vi "FFTdB&Phase_row_Ch3.vi"(8 "Freq. Step (Hz) (for Display here only)":dbl=1.0 format="%.2f", 9 "Sample Period (ms)":dbl=0.032 format="%.6f", 10 "Array Row (0base)":i16=1 min=0 max=3 step=1, 11 "Array IN":dbl[][](array[numeric]) format="%.2f") -> (0 "Phase(Radians)DataOut":dbl[](array[numeric]) format="%.2f", 1 "Magnitude( RMS dB) DataOut":dbl[](array[numeric]) format="%.2f", 2 "Magnitude (RMS dB) Plot":cluster{"Array":dbl[], "Unwrapped Phase":dbl[]}(graph), 3 "WaveformDataOut":dbl[](array[numeric]) format="%.2f", 4 "Phase (radians) Plot":cluster{"Array":dbl[], "Unwrapped Phase":dbl[]}(graph), 5 "Waveform Plot":cluster{i32, dbl, dbl[]}(graph)={0, 0.032, []})   [LabVIEW 2015]
panel:
  # "Freq. Step isn't needed if the FFT outputs are used but  the FFT-Plot outputs are not used"
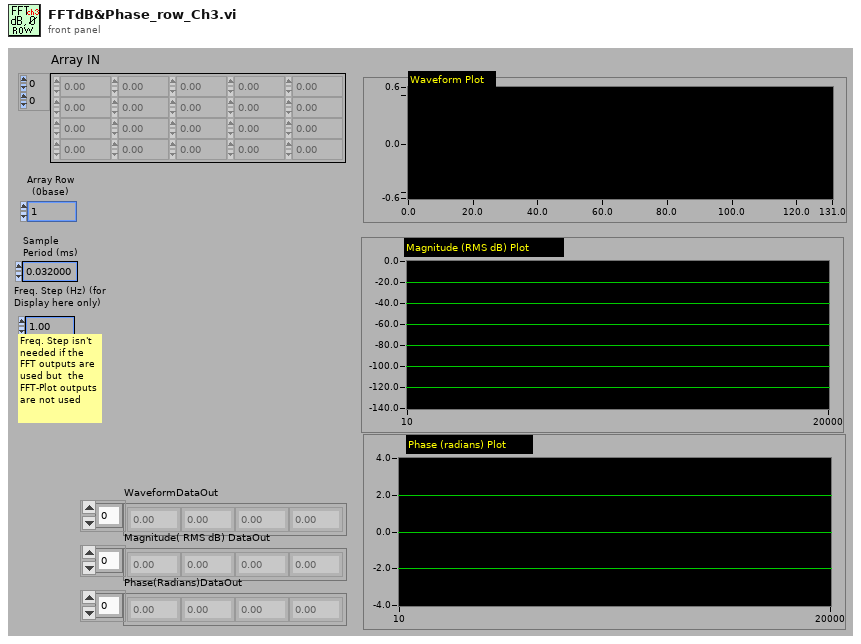
[diagram p1: front panel]
types:
  T1 = cluster{i32, "Sample Period (ms)":dbl, "Array IN":dbl[]}
  T2 = cluster{"Array":dbl[], "+Freq. Mag of FFT (dB rms)":dbl[]}
  T3 = cluster{"Array":dbl[], "+Freq Phase of FFT (radians)":dbl[]}
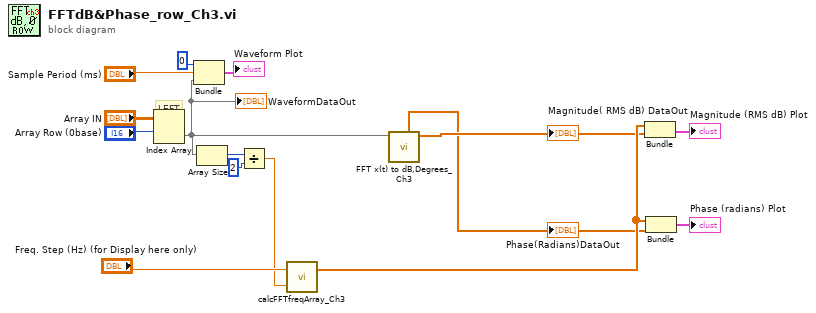
[diagram p0: block diagram]
diagram:
  # "LEFT"
  n1 = Index Array(array="Array IN", index (row)="Array Row (0base)") -> (element=w3:dbl[])  [unwired: 1 in]
  "WaveformDataOut" <- w3
  n2 = Bundle(0, "Sample Period (ms)"="Sample Period (ms)", "Array IN"=w3) -> (→"Waveform Plot":T1)  [unwired: 1 in]
  n3 = Array Size(array=w3) -> (size(s)=w7:i32)
  n4 = Divide(x=w7, y=2) -> (x/y=w6:dbl)
  n5 = call "calcFFTfreqArray_Ch3.vi"("N Freqs."=w6, "Freq. Step (Hz)"="Freq. Step (Hz) (for Display here only)") -> ("Array"=w11:dbl[])  [unwired: 1 in]
  n6 = call "FFT x(t) to dB,Degrees_Ch3.VI"("X(t)"=w3) -> ("+Freq. Mag of FFT (dB rms)"=w2:dbl[], "+Freq Phase of FFT (radians)"=w1:dbl[])  [unwired: 4 in, 5 out]
  "Magnitude( RMS dB) DataOut" <- w2
  "Phase(Radians)DataOut" <- w1
  n7 = Bundle("Array"=w11, "+Freq. Mag of FFT (dB rms)"=w2) -> (→"Magnitude (RMS dB) Plot":T2)  [unwired: 1 in]
  n8 = Bundle("Array"=w11, "+Freq Phase of FFT (radians)"=w1) -> (→"Phase (radians) Plot":T3)  [unwired: 1 in]
